vi "setUp.vi"(8 "error in (no error)":errorcluster, 11 "reference in":refnum<class "testcase-documentation.lvclass">) -> (0 "error out":errorcluster, 3 "reference out":refnum<class "testcase-documentation.lvclass">)   [LabVIEW 2017, in "testcase-documentation.lvclass"]
doc: "setUp runs prior to the test method during test execution. Use this method to initialize any object data required by your tests."
uses:
  testcase-documentation.lvclass
  C:/Program Files (x86)/National Instruments/LabVIEW 2017/vi.lib/addons/_JKI Toolkits/VI Tester/TestCase.llb/TestCase.lvclass
  testcase-documentation.lvclass/testcase-documentation.ctl
  <vilib>/addons/_JKI Toolkits/VI Tester/TestCase.llb/TestCase.lvclass
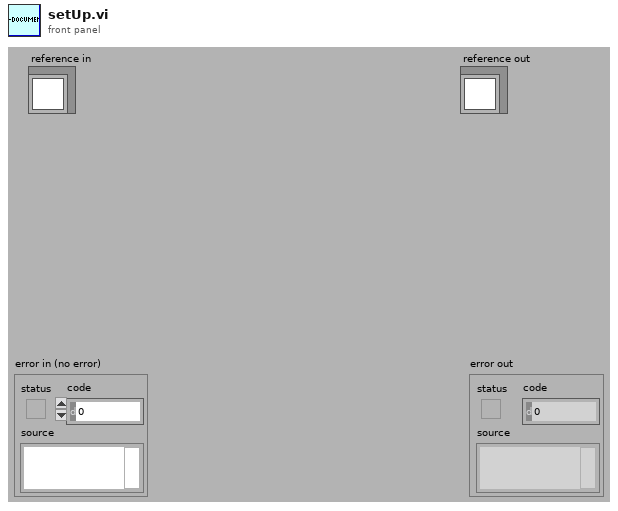
[diagram p1: front panel]
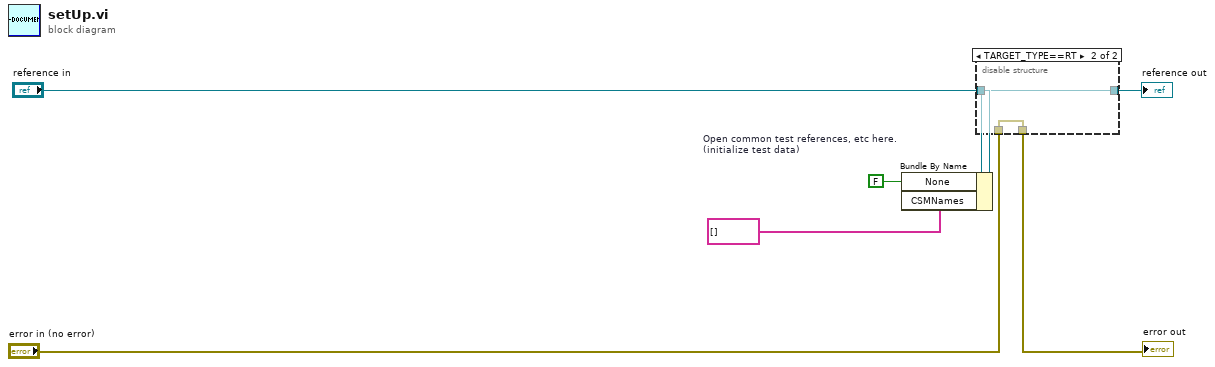
[diagram p0: block diagram]
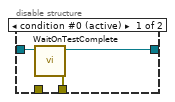
[diagram p2: hidden frame]
diagram:
  w3 = FALSE  # Open common test references, etc here. (initialize test data)
  n1 = Bundle By Name(cluster="reference in", "None"=w3, "CSMNames"=string[] []) -> (w4:refnum<class "testcase-documentation.lvclass">)
  n2 = disable-structure shown="TARGET_TYPE==RT" {
    disable-tunnel: "error in (no error)" -> [_ w11]
    disable-tunnel: [w10 w11] -> w7
    disable-tunnel: [w9 w12] -> w5
    disable-tunnel: w4 -> [w8 w12]
    frame condition #0 (active) {
      n3 = call <vilib>:"WaitOnTestComplete.vi"("TestCase in"=w8) -> ("error out"=w10:errorcluster, "TestCase out"=w9:refnum<class "testcase-documentation.lvclass">)  [unwired: 9 in]
    }
    frame condition #1 {
    }
  }
  "error out" <- w7
  "reference out" <- w5
